vi "Move Event.vi"(8 "error in (no error)":errorcluster, 9 "endIndex":i32, 10 "startIndex":i32, 11 "Tosca in":refnum<class "Parameters.lvclass">) -> (0 "error out":errorcluster, 3 "Tosca out":refnum<class "Parameters.lvclass">)   [LabVIEW 2015, in "Parameters.lvclass"]
uses:
  Parameters.lvclass
  Parameters.lvclass/Parameters.ctl
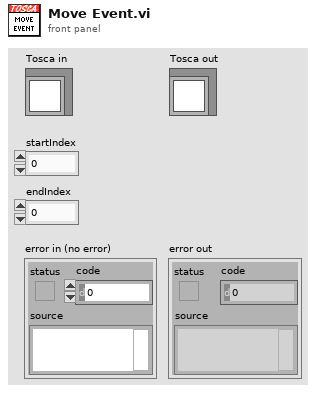
[diagram p1: front panel]
types:
  T1 = typedef "Tosca-Input Event.ctl" = cluster{"Name":string, "Criteria":T2[], "Operators":enum16{"AND", "OR"}[], "Accumulator":T4}
  T2 = typedef "Tosca-Input Criterion.ctl" = cluster{"DigInput":i32, "State":T3, "Time (ms)":i32, "Name":string}
  T3 = typedef "Logic State.ctl" = enum16{"Low", "High", "Rising", "Falling"}
  T4 = typedef "Tosca-Accumulator.ctl" = cluster{"active":bool, "N":i32, "T":dbl, "Imax":dbl, "latency":dbl}
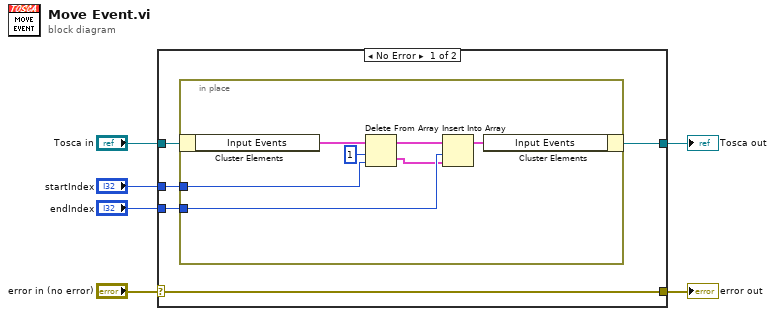
[diagram p0: block diagram]
diagram:
  n1 = case shown="No Error" "error in (no error)" {
    selector: "error in (no error)" -> [w11 w20]
    tunnel: [w11 w20] -> w5
    tunnel: [w9 w19] -> w3
    tunnel: "Tosca in" -> [w10 w19]
    tunnel: "startIndex" -> [w8 _]
    tunnel: "endIndex" -> [w7 _]
    frame No Error {
      n2 = in-place {
        in-place-border: w8 -> [w16]
        in-place-border: w7 -> [w14]
        n3 = in-place-cluster #1(w10) -> ("Input Events"=w18:T1[])
        n4 = Delete From Array(array=w18, length=1, index=w16) -> (deleted portion=w13:T1[], array with subset deleted=w15:T1[])
        n5 = Insert Into Array(array=w15, index=w14, new element=w13) -> (w12:T1[])
        n6 = in-place-cluster #1("Input Events"=w12) -> (w9:refnum<class "Parameters.lvclass">)
      }
    }
    frame Error {
    }
  }
  "error out" <- w5
  "Tosca out" <- w3
